vi "Vision Test 1.vi"(7 "error in":errorcluster) -> (20 "Matches (Pattern Matching 1)":T2(array[cluster]) {"Bounding Box"."y" format="%.2f"; "Bounding Box"."x" format="%.2f"; "Position"."y" format="%.2f"; "Position"."x" format="%.2f"; "Score" format="%.2f"; "Scale" format="%.2f"; "Angle" format="%.2f"}, 21 "Calibrated Matches (Pattern Matching 1)":T2(array[cluster]) {"Bounding Box"."y" format="%.2f"; "Bounding Box"."x" format="%.2f"; "Position"."y" format="%.2f"; "Position"."x" format="%.2f"; "Score" format="%.2f"; "Scale" format="%.2f"; "Angle" format="%.2f"}, 22 "Number of Matches (Pattern Matching 1)":i32, 27 "error out":errorcluster)   [LabVIEW 2015]
uses:
  <vilib>/vision/driver/NI_Vision_Acquisition_Software.lvlib
  <vilib>/vision/NI_Vision_Development_Module.lvlib
panel:
  out "Image Out":T1(plugin-control)
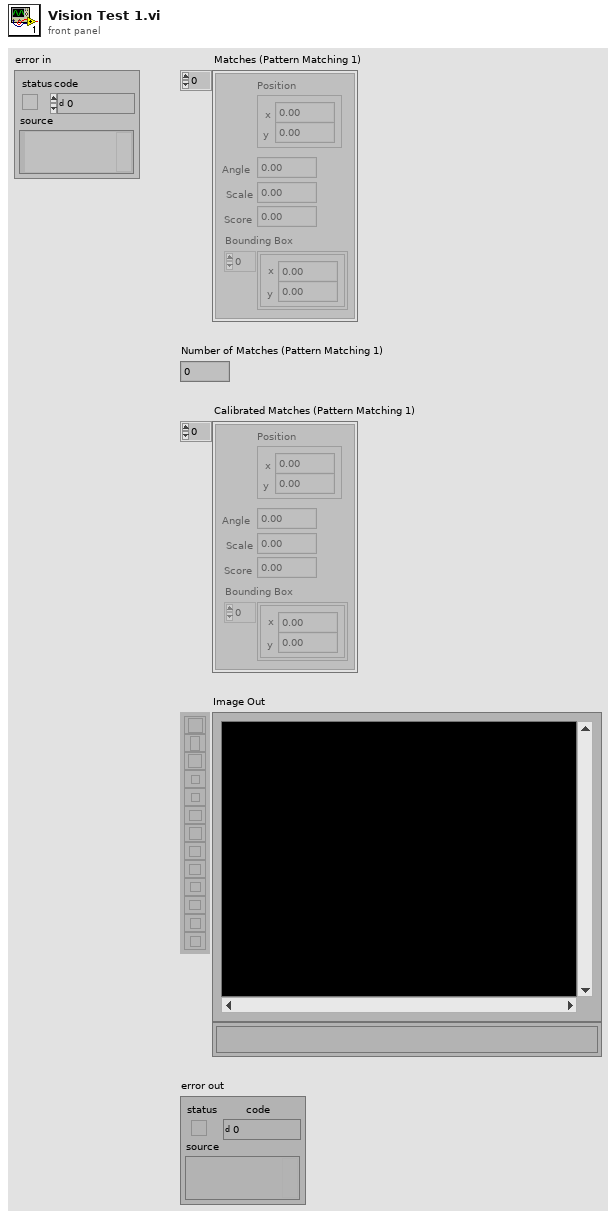
[diagram p1: front panel]
types:
  T1 = typedef "IMAQ Image.ctl" = refnum<image>
  T2 = cluster{"Position":cluster{"x":sgl, "y":sgl}, "Angle":sgl, "Scale":sgl, "Score":sgl, "Bounding Box":cluster{"x":sgl, "y":sgl}[]}[]
  T3 = cluster{"Number of Matches Requested":i32, "Minimum Match Score":sgl, "Angle Ranges":cluster{"Start Angle":sgl, "End Angle":sgl}[]}
  T4 = cluster{"Global Rectangle":i32[], "Contours":cluster{"ID":enum32{"External", "Internal"}, "Type":u32, "Coordinates":i32[]}[]}
  T5 = typedef "IMAQdx.ctl" = refnum<k21>
  T6 = cluster{"histogram":u32[], "Minimal Value":sgl, "Maximal Value":sgl, "Starting Value":sgl, "Interval Width":sgl, "Mean Value":sgl, "Standard  Variation":sgl, "Area (pixels)":i32}
  T7 = typedef "Image Type" = u32
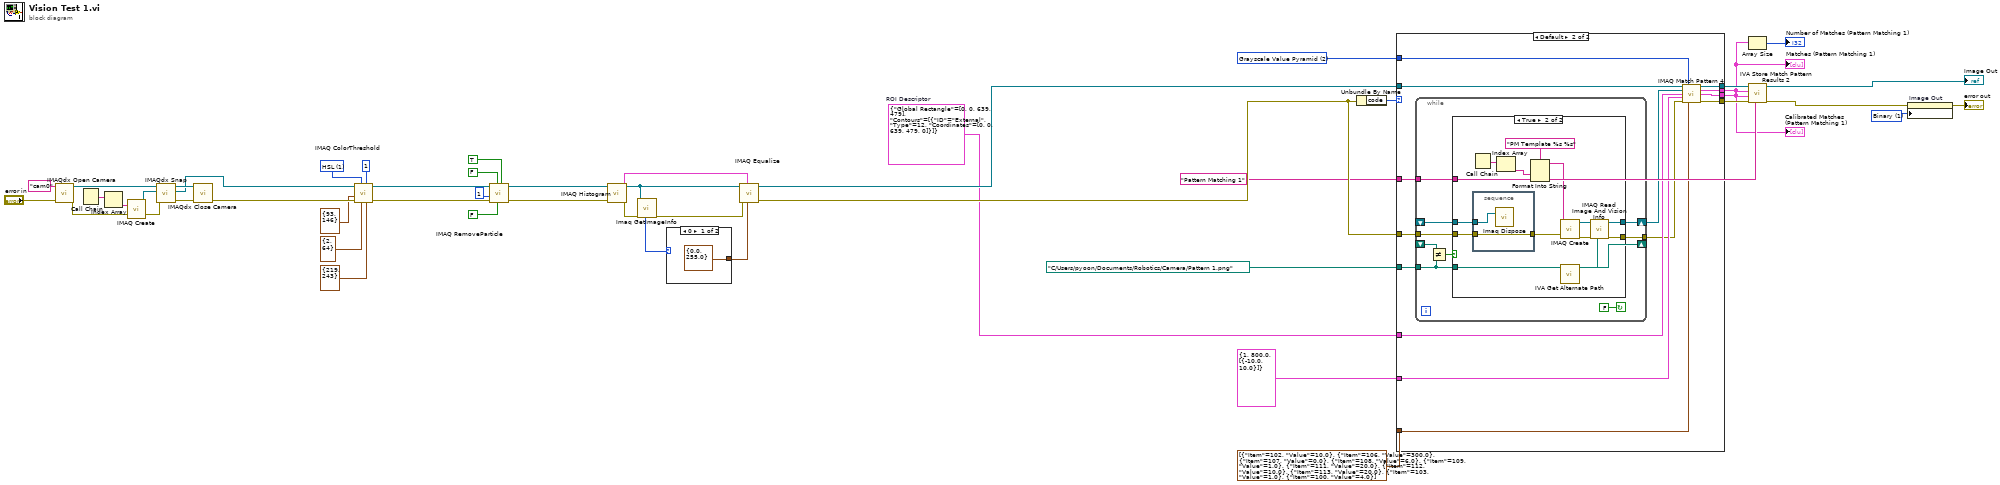
[diagram p0: block diagram]
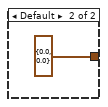
[diagram p4: hidden frame]
diagram:
  w1 = u32 1 items=["Grayscale", "Binary", "Gradient", "Rainbow", "Temperature", "User Defined", "Binary 16 Bit", "Gradient 16 Bit", "Rainbow 16 Bit", "Temperature 16 Bit", "User Defined 16 Bit"] ("Palette Type")
  w11 = 2 items=["All", "Low Discrepancy Sampling", "Grayscale Value Pyramid", "Gradients Pyramid"] ("Algorithm")
  w6 = "Pattern Matching 1" ("Step Name")
  w10 = T4 {"Global Rectangle"=[0, 0, 639, 479], "Contours"=[{"ID"=enum."External", "Type"=12, "Coordinates"=[0, 0, 639, 479, 0]}]}  # ROI Descriptor
  w36 = u16 1 items=["RGB", "HSL", "HSV", "HSI"] ("Color Mode")
  n1 = call <vilib>:"IMAQdx Open Camera.vi"("error in"="error in", "Session In"="cam0" ("Interface Name")) -> ("error out"=w47:errorcluster, "Session Out"=w41:T5)  [unwired: 1 in, 7 out]
  n2 = Call Chain() -> (call chain=w39:string[])
  n3 = Index Array(array=w39) -> (element=w38:string)  [unwired: 1 in]
  n4 = call "IMAQ Create"("Image Name"=w38, "error in (no error)"=w47) -> ("New Image"=w43:T1, "error out"=w42:errorcluster)  [unwired: 2 in, 1 out]
  n5 = call <vilib>:"IMAQdx Snap.vi"("error in"=w42, "Image In"=w43, "Session In"=w41) -> ("error out"=w45:errorcluster, "Image Out"=w32:T1, "Session Out"=w46:T5)  [unwired: 6 out]
  n6 = call <vilib>:"IMAQdx Close Camera.vi"("error in"=w45, "Session In"=w46) -> ("error out"=w44:errorcluster)  [unwired: 9 out]
  n7 = call "IMAQ ColorThreshold"("Blue or Luma or Val or Inten Range"=cluster{"Lower value":i32, "Upper value":i32} {"Lower value"=219, "Upper value"=243}, "Replace Value"=1, "Green or Sat Range"=cluster{"Lower value":i32, "Upper value":i32} {"Lower value"=2, "Upper value"=64}, "Color Mode"=w36, "error in (no error)"=w44, "Red or Hue Range"=cluster{"Lower value":i32, "Upper value":i32} {"Lower value"=93, "Upper value"=146}, "Image Src"=w32) -> ("error out"=w31:errorcluster, "Image Dst Out"=w26:T1)  [unwired: 1 in, 2 out]
  n8 = call "IMAQ RemoveParticle"("Connectivity 4/8 (8)"=TRUE, "Low Pass/High Pass (Low)"=FALSE, "Square/Hexa (Square)"=FALSE, "error in (no error)"=w31, "Number of Erosion"=1, "Image Src"=w26) -> ("error out"=w25:errorcluster, "Image Dst Out"=w21:T1)  [unwired: 1 in, 3 out]
  n9 = call "IMAQ Histogram"("error in (no error)"=w25, "Image"=w21) -> ("error out"=w20:errorcluster, "Histogram Report"=w23:T6)  [unwired: 3 in, 5 out]
  n10 = call "Imaq GetImageInfo"("error in (no error)"=w20, "Image"=w21) -> ("error out"=w19:errorcluster, "Image Type"=w22:T7)  [unwired: 8 out]
  n11 = case shown="0" w22 {
    tunnel: [cluster{"Minimum":sgl, "Maximum":sgl} {"Minimum"=0.0, "Maximum"=255.0} ("Range") cluster{"Minimum":sgl, "Maximum":sgl} {"Minimum"=0.0, "Maximum"=0.0} ("Range")] -> w18
    frame 0 {
    }
    frame Default {
    }
  }
  n12 = call "IMAQ Equalize"("Range"=w18, "Histogram Report"=w23, "error in (no error)"=w19, "Image Src"=w21) -> ("error out"=w24:errorcluster, "Image Dst Out"=w16:T1)  [unwired: 2 in, 4 out]
  n13 = Unbundle By Name(w24) -> ("code"=w12:i32)
  n14 = case shown="Default" w12 {
    tunnel: path "C:/Users/pyoon/Documents/Robotics/Camera/Pattern 1.png" ("Template File Path") -> [_ w65]
    tunnel: w24 -> [_ w64]
    tunnel: w16 -> [w51 w59]
    tunnel: [_ w60] -> w15
    tunnel: [_ w61] -> w5
    tunnel: [w51 w58] -> w13
    tunnel: w6 -> [_ w63]
    tunnel: w11 -> [_ w57]
    tunnel: w10 -> [_ w56]
    tunnel: T3 {"Number of Matches Requested"=1, "Minimum Match Score"=800.0, "Angle Ranges"=[{"Start Angle"=-10.0, "End Angle"=10.0}]} ("Parameters") -> [_ w55]
    tunnel: cluster{"Item":u16, "Value":dbl}[] [{"Item"=102, "Value"=10.0}, {"Item"=106, "Value"=300.0}, {"Item"=107, "Value"=0.0}, {"Item"=108, "Value"=6.0}, {"Item"=109, "Value"=1.0}, {"Item"=111, "Value"=20.0}, {"Item"=112, "Value"=10.0}, {"Item"=113, "Value"=20.0}, {"Item"=103, "Value"=1.0}, {"Item"=100, "Value"=4.0}] ("Advanced Options") -> [_ w53]
    tunnel: [_ w52] -> w4
    frame -1074396199, -1074396198 {
      # "Discard Coordinate System Error"
    }
    frame Default {
      n15 = while {
        shift-right: [w74] -> w62
        shift-left: _ -> [w73]
        tunnel: [w71] -> w54
        tunnel: w64 -> [w70]
        tunnel: w65 -> [w67]
        tunnel: w63 -> [w69]
        shift-right: [w67] -> _
        shift-left: _ -> [w68]
        stop <- FALSE continue-if-true
        n16 = Not Equal?(x=w68, y=w67) -> (x != y?=w66:bool)
        n17 = case shown="True" w66 {
          tunnel: [w76 w88] -> w74
          tunnel: w73 -> [w76 w79]
          tunnel: [w75 w85] -> w71
          tunnel: w70 -> [w75 w78]
          tunnel: w67 -> [_ w81]
          tunnel: w69 -> [_ w82]
          frame False {
          }
          frame True {
            n18 = stacked-sequence {
              tunnel: w79 -> [w92]
              tunnel: w78 -> [w91]
              tunnel: [w91] -> w77
              frame #0 {
                n19 = call "Imaq Dispose"("Image"=w92) -> ()  [unwired: 2 in, 4 out]
              }
            }
            n20 = Call Chain() -> (call chain=w84:string[])
            n21 = Index Array(array=w84) -> (element=w83:string)  [unwired: 1 in]
            n22 = Format Into String(format string="PM Template %s %s" ("Image Name"), w83, w82) -> (resulting string=w90:string)  [unwired: 2 in, 1 out]
            n23 = call "IMAQ Create"("Image Name"=w90, "error in (no error)"=w77) -> ("New Image"=w87:T1, "error out"=w86:errorcluster)  [unwired: 2 in, 1 out]
            n24 = call <vilib>:"IVA Get Alternate Path.vi"("Path In"=w81) -> ("Path Out"=w80:path)  [unwired: 10 out]
            n25 = call "IMAQ Read Image And Vision Info"("File Path"=w80, "error in (no error)"=w86, "Image"=w87) -> ("error out"=w85:errorcluster, "Image Out"=w88:T1)  [unwired: 1 in, 6 out]
          }
        }
      }
      n26 = call "IMAQ Match Pattern 4"("Image"=w59, "Algorithm"=w57, "Template Image"=w62, "ROI Descriptor"=w56, "Parameters"=w55, "error in (no error)"=w54, "Advanced Options"=w53) -> ("Image (duplicate)"=w58:T1, "Matches (pixel)"=w61:T2, "Matches (real-world)"=w52:T2, "error out"=w60:errorcluster)  [unwired: 4 in, 1 out]
    }
  }
  "Matches (Pattern Matching 1)" <- w5
  "Calibrated Matches (Pattern Matching 1)" <- w4
  n27 = Array Size(array=w5) -> (size(s)=→"Number of Matches (Pattern Matching 1)":i32)
  n28 = call <vilib>:"IVA Store Match Pattern Results 2.vi"("Step Name"=w6, "error in (no error)"=w15, "Matches (real-world)"=w4, "Matches (pixel)"=w5, "Image in"=w13) -> ("error out"=w14:errorcluster, "Image dup"=→"Image Out":T1)  [unwired: 1 in, 4 out]
  n29 = property on="Image Out" class="ImageControl"(error in=w14, "Palette:Palette Type"=w1) -> (error out=→"error out":errorcluster)  [unwired: 1 in, 1 out]
